vi "K2182A_Split_Cluster.vi"(0 "K2182A Cluster":T4={"Plot Window"=[], "Range"=1.0, "Update"=FALSE, "Range selector"=enum."10mV", "Auto Range"=FALSE, "V"=0.0, "Auto Range set"=FALSE}) -> (1 "K2182A Status":T3, 2 "K2182A Control":T1)   [LabVIEW 2019]
uses:
  K2812A/K2812A_cluster.ctl
  Equipment/Keithley 622x/Configure/2182 -A/Low Level/Typedefs/KE2182 -- Voltage Ranges.ctl
  K2812A/K2812A_status.ctl
  K2812A/K2812A_control.ctl
  Equipment/Keithley 622x/Keithley 622x.lvlib
panel:
  # "K 2182A"
  # "K 2182A"
  # "K 2182A"
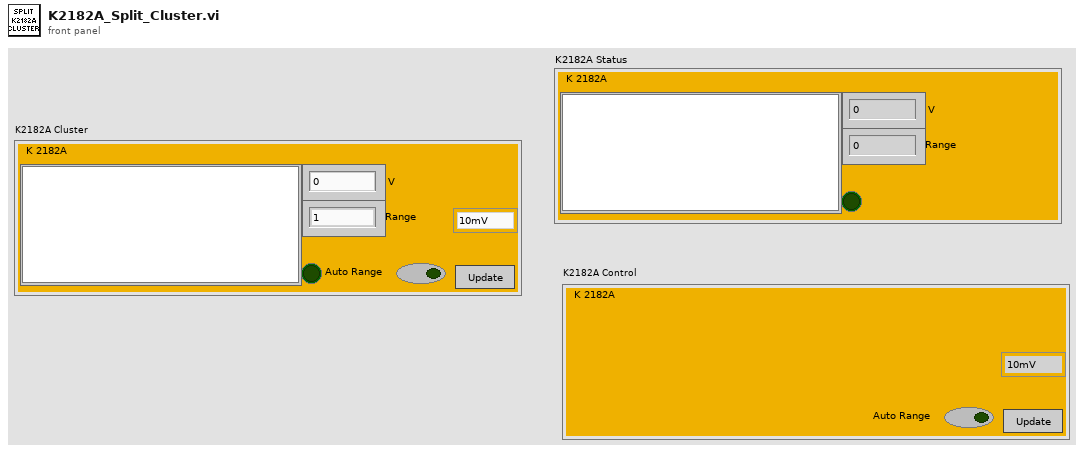
[diagram p1: front panel]
types:
  T1 = typedef "K2812A_control.ctl" = cluster{"Update":bool, "Range selector":T2, "Auto Range":bool}
  T2 = typedef "Keithley 622x.lvlib/KE2182 -- Voltage Ranges.ctl" = enum16{"10mV", "100mV", "1V", "10V", "100V"}
  T3 = typedef "K2812A_status.ctl" = cluster{"Plot Window":dbl[][], "Range":dbl, "V":dbl, "Auto Range set":bool}
  T4 = typedef "K2812A_cluster.ctl" = cluster{"Plot Window":dbl[][], "Range":dbl, "Update":bool, "Range selector":T2, "Auto Range":bool, "V":dbl, "Auto Range set":bool}
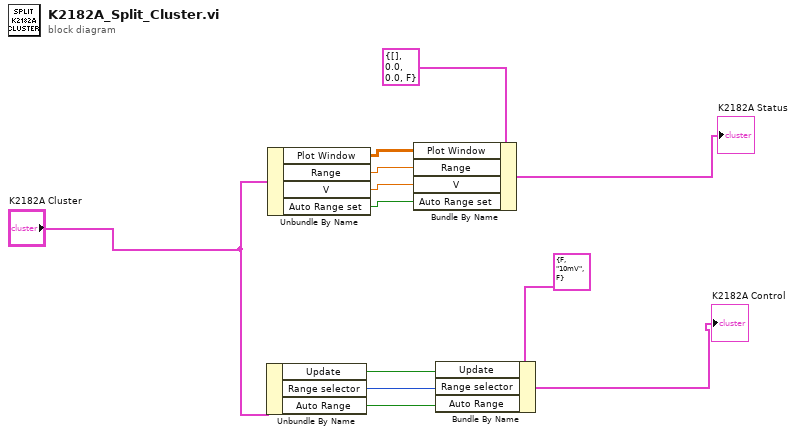
[diagram p0: block diagram]
diagram:
  n1 = Unbundle By Name("K2182A Cluster") -> ("Update"=w5:bool, "Range selector"=w6:T2, "Auto Range"=w7:bool)
  n2 = Unbundle By Name("K2182A Cluster") -> ("Plot Window"=w1:dbl[][], "Range"=w2:dbl, "V"=w3:dbl, "Auto Range set"=w4:bool)
  n3 = Bundle By Name(cluster=T3 {"Plot Window"=[], "Range"=0.0, "V"=0.0, "Auto Range set"=FALSE} ("AMI_Status 2"), "Plot Window"=w1, "Range"=w2, "V"=w3, "Auto Range set"=w4) -> (→"K2182A Status":T3)
  n4 = Bundle By Name(cluster=T1 {"Update"=FALSE, "Range selector"=enum."10mV", "Auto Range"=FALSE} ("K2182A Cluster 2"), "Update"=w5, "Range selector"=w6, "Auto Range"=w7) -> (→"K2182A Control":T1)
